vi "st_Binomial (n x).vi"(10 "x":dbl, 11 "n":i32=100) -> (0 "error":i32, 3 "binomial (n x)":dbl=0.13261955589475294)   [LabVIEW 2010, in "NI_Gmath.lvlib"]
uses:
  NI_Gmath.lvlib
  st_error_code.ctl
panel:
  # "Binomial (n x)"
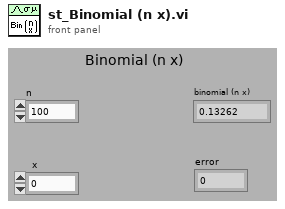
[diagram p1: front panel]
types:
  T1 = typedef "NI_Gmath.lvlib/st_error_code.ctl" = i32
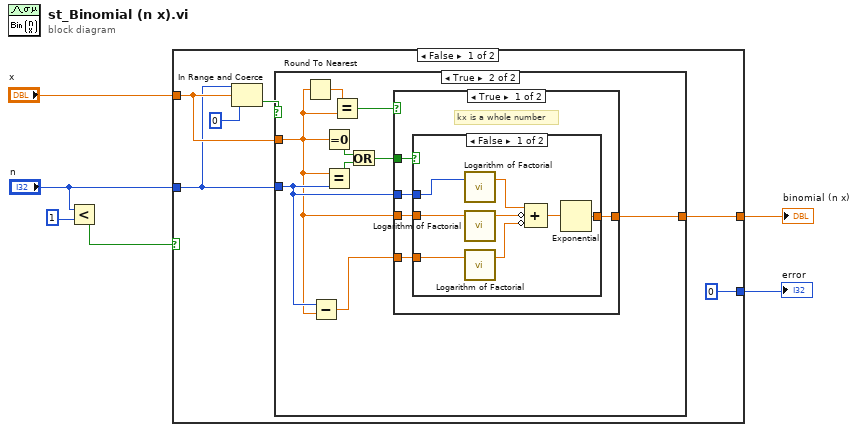
[diagram p0: block diagram]
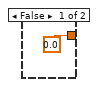
[diagram p2: hidden frame]
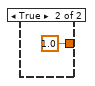
[diagram p3: hidden frame]
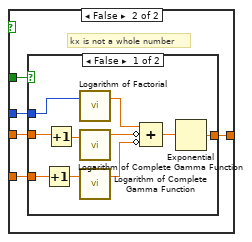
[diagram p4: hidden frame]
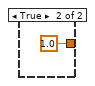
[diagram p5: hidden frame]
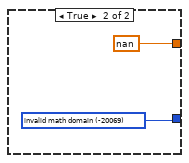
[diagram p6: hidden frame]
diagram:
  n1 = Less?(x="n", y=1) -> (x < y?=w1:bool)
  n2 = case shown="False" w1 {
    tunnel: [0 ("invalid math domain") w53] -> w6
    tunnel: [w8 nan] -> w5
    tunnel: "x" -> [w10 _]
    tunnel: "n" -> [w9 _]
    frame False {
      n3 = In Range and Coerce(upper limit=w9, x=w10, lower limit=0) -> (In Range?=w7:bool)  [unwired: 1 out]
      n4 = case shown="True" w7 {
        tunnel: [0.0 w14] -> w8
        tunnel: w10 -> [_ w17]
        tunnel: w9 -> [_ w18]
        frame False {
        }
        frame True {
          n5 = Round To Nearest(number=w17) -> (nearest integer value=w16:dbl)
          n6 = Subtract(x=w18, y=w17) -> (x-y=w20:dbl)
          n7 = Equal To 0?(x=w17) -> (x = 0?=w22:bool)
          n8 = Equal?(x=w17, y=w18) -> (x = y?=w21:bool)
          n9 = Equal?(x=w16, y=w17) -> (x = y?=w15:bool)
          n10 = Or(x=w22, y=w21) -> (x .or. y?=w19:bool)
          n11 = case shown="True" w15 {
            tunnel: w17 -> [w27 w41]
            tunnel: w20 -> [w26 w40]
            tunnel: [w25 w39] -> w14
            tunnel: w19 -> [w24 w38]
            tunnel: w18 -> [w23 w37]
            frame True {
              # "kx is a whole number"
              n12 = case shown="False" w24 {
                tunnel: w23 -> [w34 _]
                tunnel: w27 -> [w29 _]
                tunnel: w26 -> [w28 _]
                tunnel: [w32 1.0 ("t")] -> w25
                frame False {
                  n13 = call "Logarithm of Factorial.vi"("n"=w34) -> ("ln(n!)"=w35:dbl)  [unwired: 2 in]
                  n14 = call "Logarithm of Factorial.vi"("n"=w29) -> ("ln(n!)"=w31:dbl)  [unwired: 2 in]
                  n15 = call "Logarithm of Factorial.vi"("n"=w28) -> ("ln(n!)"=w30:dbl)  [unwired: 2 in]
                  n16 = Compound Arithmetic op=ADD(w35, invert w31, invert w30) -> (w33:dbl)
                  n17 = Exponential(1:w33) -> (0:w32:dbl)
                }
                frame True {
                }
              }
            }
            frame False {
              # "kx is not a whole number"
              n18 = case shown="False" w38 {
                tunnel: w37 -> [w50 _]
                tunnel: w41 -> [w47 _]
                tunnel: w40 -> [w44 _]
                tunnel: [w48 1.0 ("t")] -> w39
                frame False {
                  n19 = Increment(x=w44) -> (x+1=w43:dbl)
                  n20 = Increment(x=w47) -> (x+1=w46:dbl)
                  n21 = call "Logarithm of Factorial.vi"("n"=w50) -> ("ln(n!)"=w51:dbl)  [unwired: 2 in]
                  n22 = call "Logarithm of Complete Gamma Function.vi"("x"=w46) -> ("ln(g(x))"=w45:dbl)  [unwired: 2 in]
                  n23 = call "Logarithm of Complete Gamma Function.vi"("x"=w43) -> ("ln(g(x))"=w42:dbl)  [unwired: 2 in]
                  n24 = Compound Arithmetic op=ADD(w51, invert w45, invert w42) -> (w49:dbl)
                  n25 = Exponential(1:w49) -> (0:w48:dbl)
                }
                frame True {
                }
              }
            }
          }
        }
      }
    }
    frame True {
      w53 = T1 -20069 items=["invalid math domain"=-20069, "Fourier interpolation size m >= n"=-20070, "empty array"=-20003] ("stat interp error code")
    }
  }
  "binomial (n x)" <- w5
  "error" <- w6
